vi "DFD Integer Delay with State (Wfm).vi"(6 "state in":dbl[](array[numeric]), 8 "error in (no error)":errorcluster, 10 "delay":i32=1, 11 "signal in":waveform(dbl)={"t0"=timestamp(0 s since 1904-01-01), "dt"=0.0, "Y"=[]}) -> (0 "error out":errorcluster, 3 "signal out":waveform(dbl), 4 "state out":dbl[](array[numeric]))   [LabVIEW 2017, in "NI_DigFilterLicensed.lvlib"]
doc: "Delays a signal by a specified integer number of sample intervals. You must specify the initial internal states in the <B>state in</B> input to generate an accurate output. Wire data to the <B>signal in</B> input to determine the polymorphic instance to use or manually select the instance."
uses:
  <vilib>/addons/Digital Filter Design/NI_DigFilterLicensed.lvlib
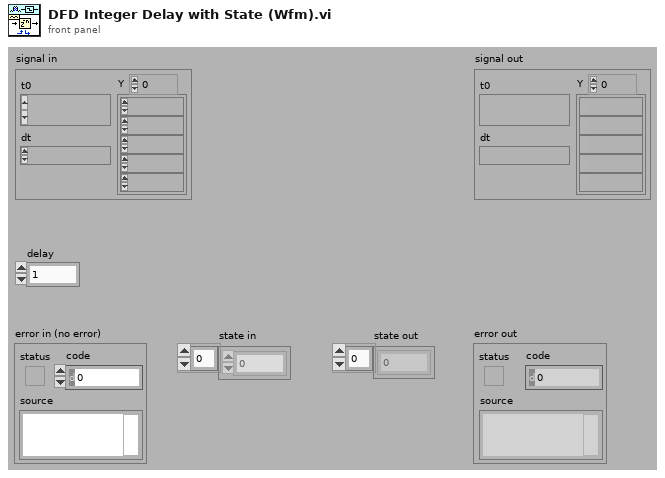
[diagram p1: front panel]
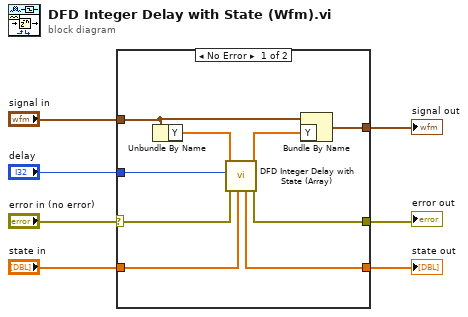
[diagram p0: block diagram]
diagram:
  n1 = case shown="No Error" "error in (no error)" {
    selector: "error in (no error)" -> [w12 w17]
    tunnel: [w11 w17] -> w6
    tunnel: "state in" -> [w15 _]
    tunnel: "delay" -> [w16 _]
    tunnel: "signal in" -> [w10 _]
    tunnel: [w14 _] -> w2
    tunnel: [w13 _] -> w1
    frame No Error {
      n2 = Unbundle By Name(w10) -> ("Y"=w9:dbl[])
      n3 = call <vilib>:"DFD Integer Delay with State (Array).vi"("state in"=w15, "error in (no error)"=w12, "delay"=w16, "signal in"=w9) -> ("error out"=w11:errorcluster, "signal out"=w8:dbl[], "state out"=w14:dbl[])  [unwired: 5 out]
      n4 = Bundle By Name(cluster=w10, "Y"=w8) -> (w13:waveform(dbl))
    }
    frame Error {
    }
  }
  "error out" <- w6
  "signal out" <- w1
  "state out" <- w2
